vi "VolumeMaster 2012 NIVerified.vi"() -> ()   [LabVIEW 2012]
uses:
  <vilib>/Utility/inputDevices.llb/keyboardAcquire.vi
  <vilib>/Utility/inputDevices.llb/closeKeyboard.vi
panel:
  in  "Cancel Button":bool
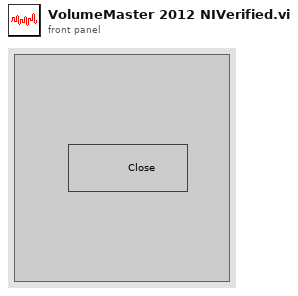
[diagram p1: front panel]
types:
  T1 = enum16{"0", "1", "2", "3", "4", "5", "6", "7", "8", "9", "A", "B", "C", "D", "E", "F", "G", "H", "I", "J", "K", "L", "M", "N", "O", "P", "Q", "R", "S", "T", "U", "V", "W", "X", "Y", "Z", "F1", "F2", "F3", "F4", "F5", "F6", "F7", "F8", "F9", "F10", "F11", "F12", "F13", "F14", "F15", "ADD", "BACK", "BACKSLASH", "CAPITAL", "COMMA", "DECIMAL", "DELETE", "DIVIDE", "DOWN", "END", "EQUALS", "ESCAPE", "GRAVE (`)", "HOME", "INSERT", "LBRACKET", "LCONTROL", "LEFT", "L ALT", "LSHIFT", "LWIN", "MINUS", "MULTIPLY", "NEXT", "NUMLOCK", "NUMPAD_0", "NUMPAD_1", "NUMPAD_2", "NUMPAD_3", "NUMPAD_4", "NUMPAD_5", "NUMPAD_6", "NUMPAD_7", "NUMPAD_8", "NUMPAD_9", "PAUSE", "PERIOD", "PRIOR (PG UP)", "RBRACKET", "RCONTROL", "RETURN", "RIGHT", "R ALT", "RSHIFT", "RWIN", "SCROLL", "SEMICOLON", "SLASH", "SPACE", "SUBTRACT", "TAB", "UP", "ENTER (num pad)", "' (quote)"}[]
  T2 = enum16{"0", "1", "2", "3", "4", "5", "6", "7", "8", "9", "A", "B", "C", "D", "E", "F", "G", "H", "I", "J", "K", "L", "M", "N", "O", "P", "Q", "R", "S", "T", "U", "V", "W", "X", "Y", "Z", "F1", "F2", "F3", "F4", "F5", "F6", "F7", "F8", "F9", "F10", "F11", "F12", "F13", "F14", "F15", "ADD", "BACK", "BACKSLASH", "CAPITAL", "COMMA", "DECIMAL", "DELETE", "DIVIDE", "DOWN", "END", "EQUALS", "ESCAPE", "GRAVE (`)", "HOME", "INSERT", "LBRACKET", "LCONTROL", "LEFT", "L ALT", "LSHIFT", "LWIN", "MINUS", "MULTIPLY", "NEXT", "NUMLOCK", "NUMPAD_0", "NUMPAD_1", "NUMPAD_2", "NUMPAD_3", "NUMPAD_4", "NUMPAD_5", "NUMPAD_6", "NUMPAD_7", "NUMPAD_8", "NUMPAD_9", "PAUSE", "PERIOD", "PRIOR (PG UP)", "RBRACKET", "RCONTROL", "RETURN", "RIGHT", "R ALT", "RSHIFT", "RWIN", "SCROLL", "SEMICOLON", "SLASH", "SPACE", "SUBTRACT", "TAB", "UP", "ENTER (num pad)", "' (quote)"}
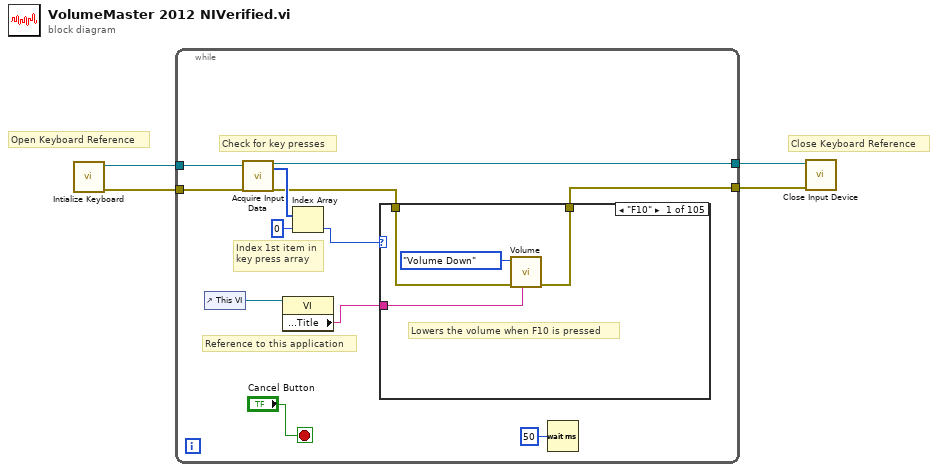
[diagram p0: block diagram]
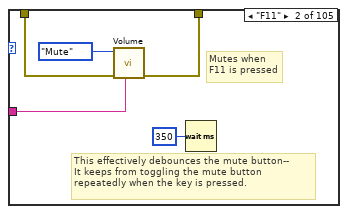
[diagram p2: hidden frame]
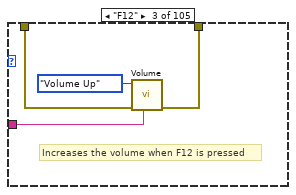
[diagram p3: hidden frame]
diagram:
  # "Close Keyboard Reference"
  # "Open Keyboard Reference"
  n1 = call <vilib>:"Intialize Keyboard.vi"() -> ("error out"=w3:errorcluster, "device ID"=w4:refnum<k1>)  [unwired: 10 in]
  n2 = while {
    tunnel: w4 -> [w16]
    tunnel: w3 -> [w15]
    tunnel: [w11] -> w2
    tunnel: [w9] -> w1
    stop <- "Cancel Button" stop-if-true
    # "Reference to this application"
    # "Index 1st item in\nkey press array"
    # "Check for key presses"
    n3 = control-ref of="This VI"() -> (w6:refnum<vi>)
    n4 = call-poly <vilib>:"Acquire Input Data.vi"("device ID"=w16, "error in (no error)"=w15) -> ("device ID"=w11:refnum<k1>, "keys pressed"=w14:T1, "error out"=w10:errorcluster)  [unwired: 15 in]
    n5 = property class="VI"(reference=w6) -> ("Front Panel.Title"=w5:string)  [unwired: 1 in, 2 out]
    n6 = Index Array(array=w14, index=0) -> (element=w8:T2)
    n7 = case shown="\"F10\"" w8 {
      tunnel: w10 -> [w19 w24 w28 w30 w31 w32 w33 w34 w35 w36 w37 w38 w39 w40 w41 w42 w43 w44 w45 w46 w47 w48 w49 w50 w51 w52 w53 w54 w55 w56 w57 w58 w59 w60 w61 w62 w63 w64 w65 w66 w67 w68 w69 w70 w71 w72 w73 w74 w75 w76 w77 w78 w79 w80 w81 w82 w83 w84 w85 w86 w87 w88 w89 w90 w91 w92 w93 w94 w95 w96 w97 w98 w99 w100 w101 w102 w103 w104 w105 w106 w107 w108 w109 w110 w111 w112 w113 w114 w115 w116 w117 w118 w119 w120 w121 w122 w123 w124 w125 w126 w127 w128 w129 w130 w131]
      tunnel: [w18 w23 w27 w30 w31 w32 w33 w34 w35 w36 w37 w38 w39 w40 w41 w42 w43 w44 w45 w46 w47 w48 w49 w50 w51 w52 w53 w54 w55 w56 w57 w58 w59 w60 w61 w62 w63 w64 w65 w66 w67 w68 w69 w70 w71 w72 w73 w74 w75 w76 w77 w78 w79 w80 w81 w82 w83 w84 w85 w86 w87 w88 w89 w90 w91 w92 w93 w94 w95 w96 w97 w98 w99 w100 w101 w102 w103 w104 w105 w106 w107 w108 w109 w110 w111 w112 w113 w114 w115 w116 w117 w118 w119 w120 w121 w122 w123 w124 w125 w126 w127 w128 w129 w130 w131] -> w9
      tunnel: w5 -> [w17 w21 w26 _ _ _ _ _ _ _ _ _ _ _ _ _ _ _ _ _ _ _ _ _ _ _ _ _ _ _ _ _ _ _ _ _ _ _ _ _ _ _ _ _ _ _ _ _ _ _ _ _ _ _ _ _ _ _ _ _ _ _ _ _ _ _ _ _ _ _ _ _ _ _ _ _ _ _ _ _ _ _ _ _ _ _ _ _ _ _ _ _ _ _ _ _ _ _ _ _ _ _ _ _ _]
      frame "F10" {
        # "Lowers the volume when F10 is pressed"
        n8 = call "Volume.vi"("lpszWindowName"=w17, "error in (no error)"=w19, "Enum"=enum16{"Mute", "Volume Up", "Volume Down"}."Volume Down") -> ("error out"=w18:errorcluster)  [unwired: 8 in]
      }
      frame "F11" {
        # "Mutes when\nF11 is pressed"
        # "This effectively debounces the mute button--\nIt keeps from toggling the mute button\nrepeatedly when the key is pressed."
        n9 = call "Volume.vi"("lpszWindowName"=w21, "error in (no error)"=w24, "Enum"=enum16{"Mute", "Volume Up", "Volume Down"}."Mute") -> ("error out"=w23:errorcluster)  [unwired: 8 in]
        n10 = Wait (ms)(milliseconds to wait=u32 350) -> ()  [unwired: 1 out]
      }
      frame "F12" {
        # "Increases the volume when F12 is pressed"
        n11 = call "Volume.vi"("lpszWindowName"=w26, "error in (no error)"=w28, "Enum"=enum16{"Mute", "Volume Up", "Volume Down"}."Volume Up") -> ("error out"=w27:errorcluster)  [unwired: 8 in]
      }
      frame "F13" {
      }
      frame "F14" {
      }
      frame "F15" {
      }
      frame "ADD" {
      }
      frame "BACK" {
      }
      frame "BACKSLASH" {
      }
      frame "CAPITAL" {
      }
      frame "COMMA" {
      }
      frame "DECIMAL" {
      }
      frame "DELETE" {
      }
      frame "DIVIDE" {
      }
      frame "DOWN" {
      }
      frame "END" {
      }
      frame "EQUALS" {
      }
      frame "ESCAPE" {
      }
      frame "GRAVE (`)" {
      }
      frame "HOME" {
      }
      frame "INSERT" {
      }
      frame "LBRACKET" {
      }
      frame "LCONTROL" {
      }
      frame "LEFT" {
      }
      frame "L ALT" {
      }
      frame "LSHIFT" {
      }
      frame "LWIN" {
      }
      frame "MINUS" {
      }
      frame "MULTIPLY" {
      }
      frame "NEXT" {
      }
      frame "NUMLOCK" {
      }
      frame "NUMPAD_0" {
      }
      frame "NUMPAD_1" {
      }
      frame "NUMPAD_2" {
      }
      frame "NUMPAD_3" {
      }
      frame "NUMPAD_4" {
      }
      frame "NUMPAD_5" {
      }
      frame "NUMPAD_6" {
      }
      frame "NUMPAD_7" {
      }
      frame "NUMPAD_8" {
      }
      frame "NUMPAD_9" {
      }
      frame "PAUSE" {
      }
      frame "PERIOD" {
      }
      frame "PRIOR (PG UP)" {
      }
      frame "RBRACKET" {
      }
      frame "RCONTROL" {
      }
      frame "RETURN" {
      }
      frame "RIGHT" {
      }
      frame "R ALT" {
      }
      frame "RSHIFT" {
      }
      frame "RWIN" {
      }
      frame "SCROLL" {
      }
      frame "SEMICOLON" {
      }
      frame "SLASH" {
      }
      frame "SPACE" {
      }
      frame "SUBTRACT" {
      }
      frame "TAB" {
      }
      frame "UP" {
      }
      frame "ENTER (num pad)" {
      }
      frame "' (quote)" {
      }
      frame "F9" {
      }
      frame "F8" {
      }
      frame "F7" {
      }
      frame "F6" {
      }
      frame "F5" {
      }
      frame "F4" {
      }
      frame "F3" {
      }
      frame "F2" {
      }
      frame "F1" {
      }
      frame "Z" {
      }
      frame "Y" {
      }
      frame "X" {
      }
      frame "W" {
      }
      frame "V" {
      }
      frame "U" {
      }
      frame "T" {
      }
      frame "S" {
      }
      frame "R" {
      }
      frame "Q" {
      }
      frame "P" {
      }
      frame "O" {
      }
      frame "N" {
      }
      frame "M" {
      }
      frame "L" {
      }
      frame "K" {
      }
      frame "J" {
      }
      frame "I" {
      }
      frame "H" {
      }
      frame "G" {
      }
      frame "F" {
      }
      frame "E" {
      }
      frame "D" {
      }
      frame "C" {
      }
      frame "B" {
      }
      frame "A" {
      }
      frame "9" {
      }
      frame "8" {
      }
      frame "7" {
      }
      frame "6" {
      }
      frame "5" {
      }
      frame "4" {
      }
      frame "3" {
      }
      frame "2" {
      }
      frame "1" {
      }
      frame "0" {
      }
    }
    n12 = Wait (ms)(milliseconds to wait=u32 50) -> ()  [unwired: 1 out]
  }
  n13 = call-poly <vilib>:"Close Input Device.vi"("error in (no error)"=w1, "device ID"=w2) -> ()  [unwired: 8 in, 1 out]
